vi "A131258.vi"() -> ()   [LabVIEW 2020]
panel:
  in  "轴承压装力位移曲线":refnum<vi>
  in  "最大压销力":dbl
  in  "右泄露":dbl
  in  "左泄露":dbl
  in  "逆向8":dbl
  in  "正向8":dbl
  in  "逆向5":dbl
  in  "正向5":dbl
  in  "逆向3":dbl
  in  "正向3":dbl
  in  "逆向1":dbl
  in  "正向1":dbl
  in  "对称性全":dbl
  in  "对称性5":dbl
  in  "对称性1":dbl
  in  "定点C":dbl
  in  "力特性":T1
  in  "力位移曲线":refnum<vi>
  in  "LED-力位移":refnum<vi>
  in  "定点B":dbl
  in  "定点A":dbl
  in  "压力损失":cluster{"下限":dbl, "上限":dbl}
  in  "灵敏度":T2
  in  "内泄露曲线":refnum<vi>
  in  "压销力":cluster{"下限":dbl, "上限":dbl}
  in  "LED-自由间隙":refnum<vi>
  in  "LED-内泄露":refnum<vi>
  in  "LED-灵敏度":refnum<vi>
  in  "LED-力特性":refnum<vi>
  in  "内泄露":cluster{"下限":dbl, "上限":dbl}
  in  "试验项":enum32{"力特性", "压销位移力曲线"}(tab)
  in  "力特性曲线":refnum<vi>
  in  "自由间隙曲线":refnum<vi>
  in  "灵敏度曲线":refnum<vi>
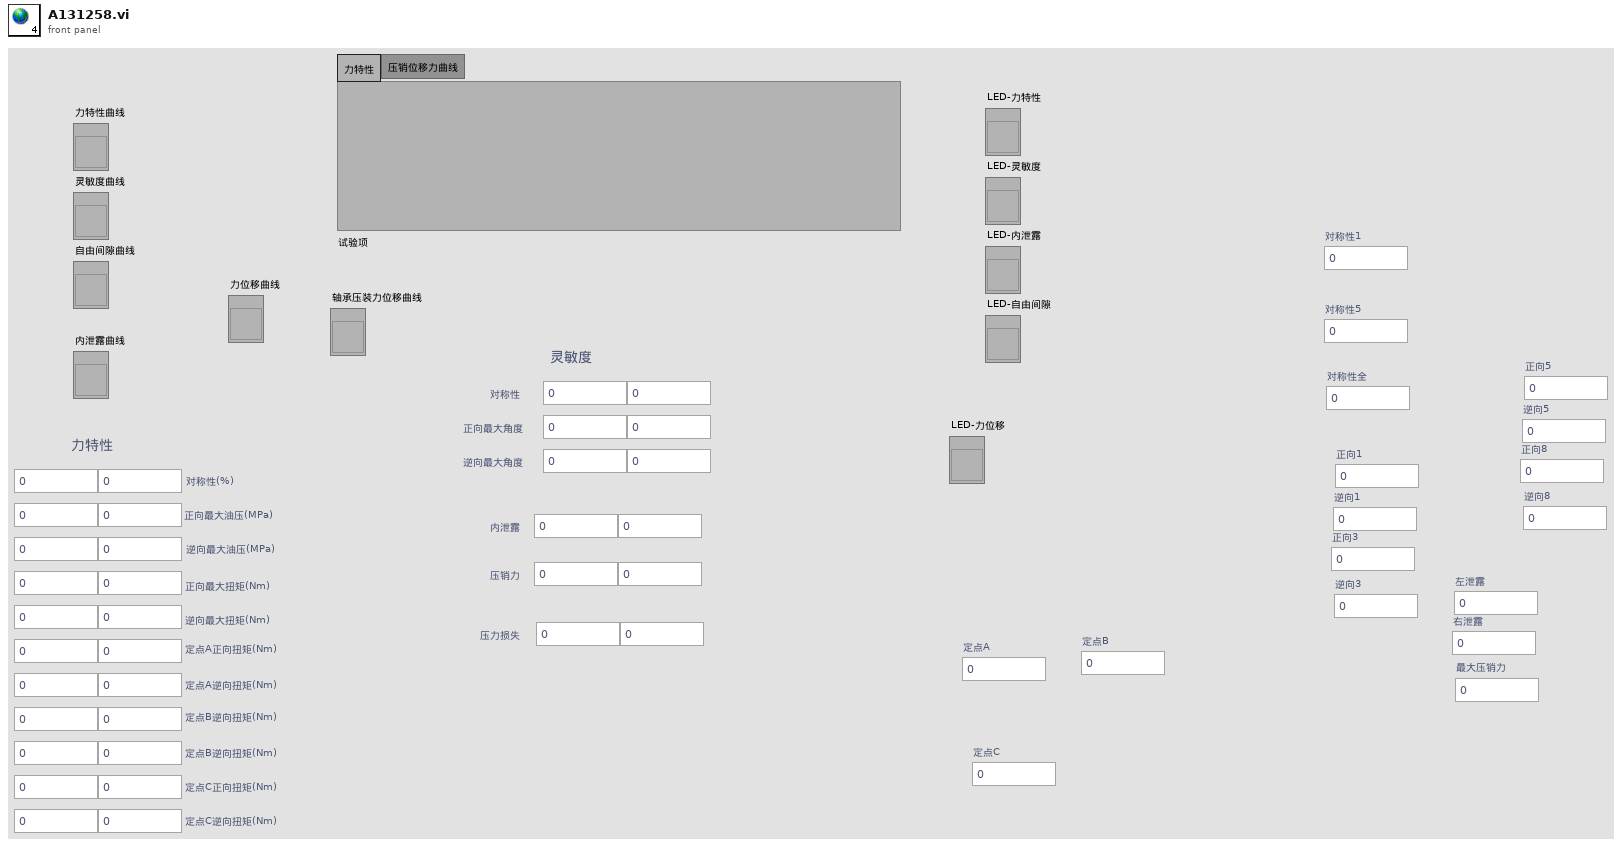
[diagram p1: front panel]
types:
  T1 = cluster{"对称性(%)":cluster{"下限":dbl, "上限":dbl}, "正向最大油压(MPa)":cluster{"下限":dbl, "上限":dbl}, "逆向最大油压(MPa)":cluster{"下限":dbl, "上限":dbl}, "正向最大扭矩(Nm)":cluster{"下限":dbl, "上限":dbl}, "逆向最大扭矩(Nm)":cluster{"上限":dbl, "下限":dbl}, "定点A正向扭矩(Nm)":cluster{"下限":dbl, "上限":dbl}, "定点A逆向扭矩(Nm)":cluster{"下限":dbl, "上限":dbl}, "定点B逆向扭矩(Nm)":cluster{"下限":dbl, "上限":dbl}, "定点B逆向扭矩(Nm)":cluster{"下限":dbl, "上限":dbl}, "定点C正向扭矩(Nm)":cluster{"下限":dbl, "上限":dbl}, "定点C逆向扭矩(Nm)":cluster{"下限":dbl, "上限":dbl}}
  T2 = cluster{"         对称性":cluster{"下限":dbl, "上限":dbl}, "正向最大角度":cluster{"下限":dbl, "上限":dbl}, "逆向最大角度":cluster{"下限":dbl, "上限":dbl}}
diagram:
